vi "Creating a SubVI.vi"() -> ()   [LabVIEW 2010]
doc: "This VI demonstrates where to use subVIs to perform repeated calculations."
panel:
  in  "Function 3":cluster{"a":dbl, "b":dbl, "c":dbl, "d":dbl}
  in  "Function 2":cluster{"a":dbl, "b":dbl, "c":dbl, "d":dbl}
  in  "Function 1":cluster{"a":dbl, "b":dbl, "c":dbl, "d":dbl}
  out "XY Graph":cluster{i32[], dbl[]}[](graph)
  in  "Ending x value":i32=100
  in  "Starting x value":i32=-100
  # "ax^3+bx^2+cx+d"
  # "Domain"
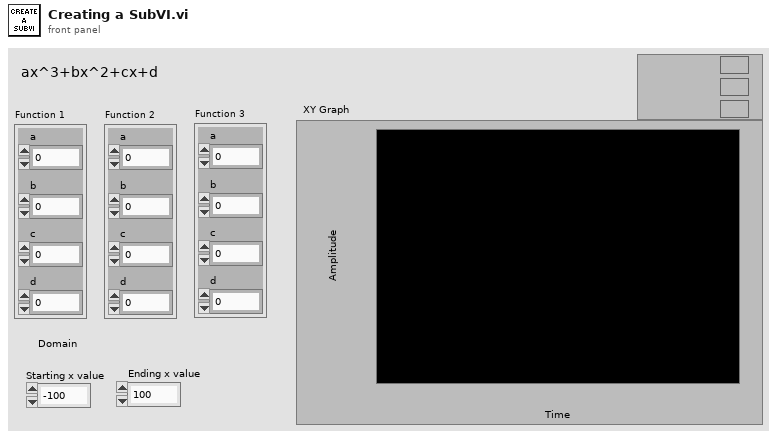
[diagram p1: front panel]
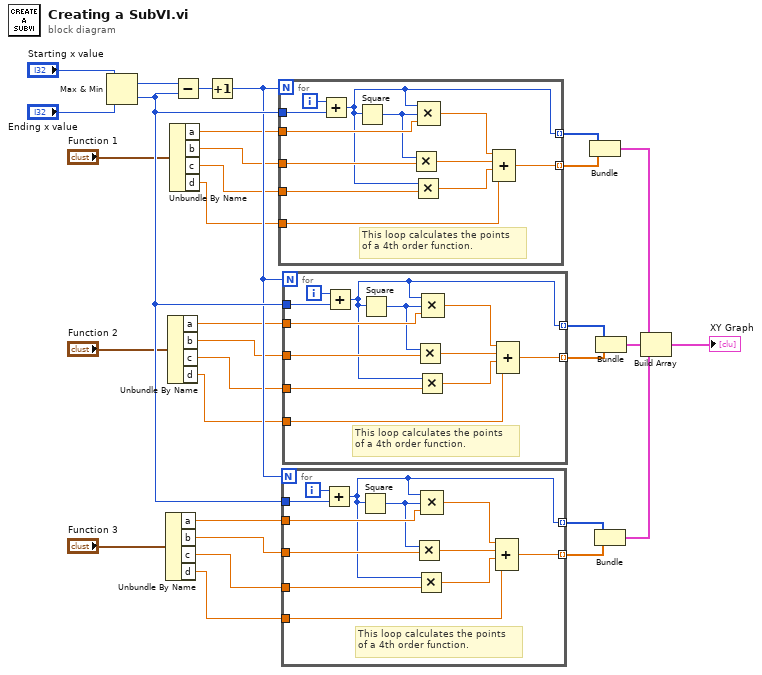
[diagram p0: block diagram]
diagram:
  n1 = Max & Min(x="Starting x value", y="Ending x value") -> (max(x,y)=w29:i32, min(x,y)=w21:i32)
  n2 = Unbundle By Name("Function 3") -> ("a"=w5:dbl, "b"=w4:dbl, "c"=w3:dbl, "d"=w2:dbl)
  n3 = Unbundle By Name("Function 2") -> ("a"=w10:dbl, "b"=w8:dbl, "c"=w7:dbl, "d"=w6:dbl)
  n4 = Unbundle By Name("Function 1") -> ("a"=w14:dbl, "b"=w13:dbl, "c"=w12:dbl, "d"=w11:dbl)
  n5 = Subtract(x=w29, y=w21) -> (x-y=w28:i32)
  n6 = Increment(x=w28) -> (x+1=w20:i32)
  n7 = for {
    N: w20 -> [_]
    tunnel: w14 -> [w43]
    tunnel: w13 -> [w41]
    tunnel: w12 -> [w40]
    tunnel: w11 -> [w36]
    tunnel: [w35] -> w27 mode=indexing
    tunnel: [w34] -> w26 mode=indexing
    tunnel: w21 -> [w33]
    i -> [w32]
    # "This loop calculates the points \nof a 4th order function."
    n8 = Add(x=w32, y=w33) -> (x+y=w34:i32)
    n9 = Square(x=w34) -> (x^2=w42:i32)
    n10 = Multiply(x=w42, y=w41) -> (x*y=w38:dbl)
    n11 = Multiply(x=w34, y=w40) -> (x*y=w39:dbl)
    n12 = Compound Arithmetic op=MULTIPLY(w34, w42, w43) -> (w37:dbl)
    n13 = Compound Arithmetic op=ADD(w37, w38, w39, w36) -> (w35:dbl)
  }
  n14 = for {
    N: w20 -> [_]
    tunnel: w5 -> [w55]
    tunnel: w4 -> [w53]
    tunnel: w3 -> [w52]
    tunnel: w2 -> [w48]
    tunnel: [w47] -> w18 mode=indexing
    tunnel: [w46] -> w19 mode=indexing
    tunnel: w21 -> [w45]
    i -> [w44]
    # "This loop calculates the points \nof a 4th order function."
    n15 = Add(x=w44, y=w45) -> (x+y=w46:i32)
    n16 = Square(x=w46) -> (x^2=w54:i32)
    n17 = Multiply(x=w54, y=w53) -> (x*y=w50:dbl)
    n18 = Multiply(x=w46, y=w52) -> (x*y=w51:dbl)
    n19 = Compound Arithmetic op=MULTIPLY(w46, w54, w55) -> (w49:dbl)
    n20 = Compound Arithmetic op=ADD(w49, w50, w51, w48) -> (w47:dbl)
  }
  n21 = for {
    N: w20 -> [_]
    tunnel: w10 -> [w67]
    tunnel: w8 -> [w65]
    tunnel: w7 -> [w64]
    tunnel: w6 -> [w60]
    tunnel: [w59] -> w17 mode=indexing
    tunnel: [w58] -> w16 mode=indexing
    tunnel: w21 -> [w57]
    i -> [w56]
    # "This loop calculates the points \nof a 4th order function."
    n22 = Add(x=w56, y=w57) -> (x+y=w58:i32)
    n23 = Square(x=w58) -> (x^2=w66:i32)
    n24 = Multiply(x=w66, y=w65) -> (x*y=w62:dbl)
    n25 = Multiply(x=w58, y=w64) -> (x*y=w63:dbl)
    n26 = Compound Arithmetic op=MULTIPLY(w58, w66, w67) -> (w61:dbl)
    n27 = Compound Arithmetic op=ADD(w61, w62, w63, w60) -> (w59:dbl)
  }
  n28 = Bundle(w26, w27) -> (w25:cluster{i32[], dbl[]})  [unwired: 1 in]
  n29 = Bundle(w19, w18) -> (w23:cluster{i32[], dbl[]})  [unwired: 1 in]
  n30 = Bundle(w16, w17) -> (w24:cluster{i32[], dbl[]})  [unwired: 1 in]
  n31 = Build Array(w25, w24, w23) -> (→"XY Graph":cluster{i32[], dbl[]}[])
